vi "RSNRPZ Set Scope Offset Time.vi"(8 "error in (no error)":errorcluster, 9 "Offset Time (0.0)":dbl format="%.2p", 10 "Channel (1)":i32=1, 11 "VISA session":refnum<visa-resource-name> caption="VISA resource name") -> (0 "error out":errorcluster, 3 "dup VISA session":refnum<visa-resource-name> caption="VISA resource name")   [LabVIEW 2010]
doc: "This VI determines the relative position of the trigger event in relation to the beginning of the Scope measurement sequence.\n\nNote:\n\n1) This VI is not available for NRP-Z51.\n\nRemote-control command(s):\nSENS:TRAC:OFFS:TIME"
uses:
  rsnrpz_32.dll
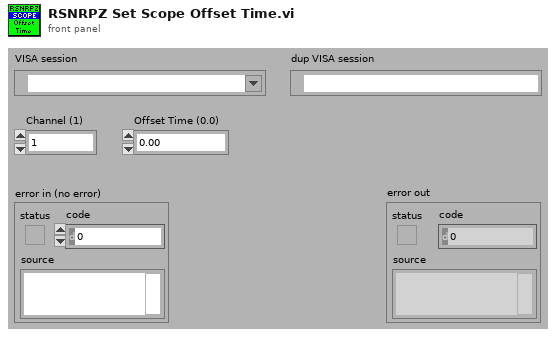
[diagram p1: front panel]
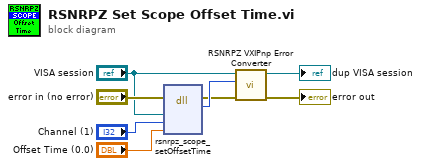
[diagram p0: block diagram]
diagram:
  n1 = dll-call lib="rsnrpz_32.dll" fn="rsnrpz_scope_setOffsetTime"(error in="error in (no error)", "VISA Session"="VISA session", "Channel"="Channel (1)", "Offset Time"="Offset Time (0.0)") -> (error out=w5:errorcluster, "Status"=w8:i32)  [unwired: 5 in, 1 out]
  n2 = call <instrlib>:"RSNRPZ VXIPnp Error Converter.vi"("error in"=w5, "VXIPnp error code"=w8, "VISA session"="VISA session") -> ("error out"=→"error out":errorcluster, "dup VISA session"=→"dup VISA session":refnum<visa-resource-name>)  [unwired: 7 in]
